vi "Edit Structure.vi"(4 "EOH":u8, 5 "Edit structure":bool, 6 "No. of Bytes":u16, 7 "Channel ID":enum16{""}(ring), 8 "Message ID":u8, 9 "SOH":u8, 11 "MulticolumnListbox in":refnum<vi>) -> ()   [LabVIEW 2020]
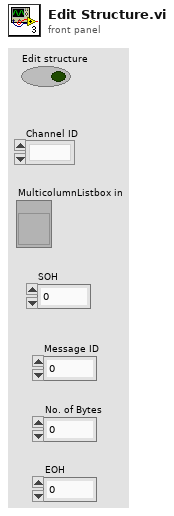
[diagram p1: front panel]
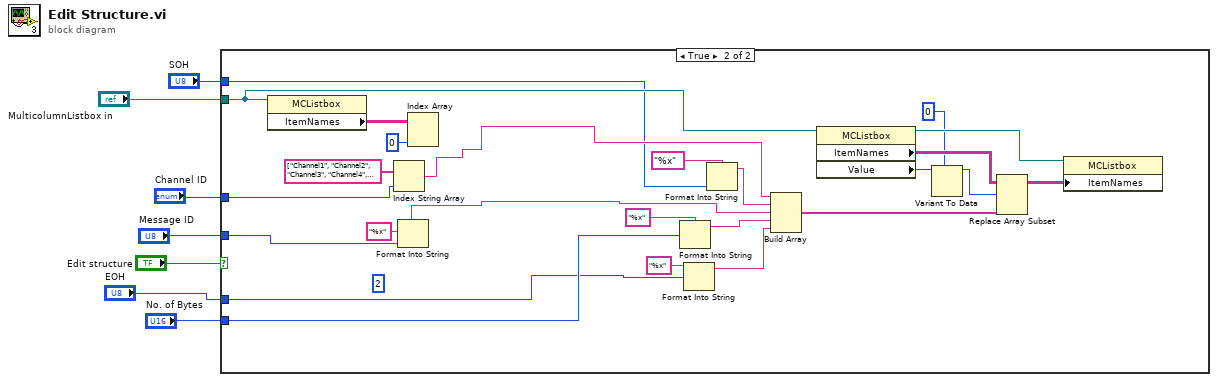
[diagram p0: block diagram]
diagram:
  n1 = case shown="True" "Edit structure" {
    tunnel: "MulticolumnListbox in" -> [_ w27]
    tunnel: "Channel ID" -> [_ w22]
    tunnel: "Message ID" -> [_ w21]
    tunnel: "SOH" -> [_ w25]
    tunnel: "No. of Bytes" -> [_ w24]
    tunnel: "EOH" -> [_ w23]
    frame False {
    }
    frame True {
      (unwired) 2 ("disabled index (col)")
      n2 = property class="MCListbox"(reference=w27) -> ("ItemNames"=w30:string[][])  [unwired: 1 in, 2 out]
      n3 = Index String Array(1:w22, 2:string[] ["Channel1", "Channel2", "Channel3", "Channel4", "Channel5", "Channel6", "Channel7", "Channel8"] ("string array")) -> (0:w29:string)  [unwired: 1 in]
      n4 = Format Into String(format string="%x", w21) -> (resulting string=w28:string)  [unwired: 2 in, 1 out]
      n5 = Index Array(array=w30, index (col)=0 ("disabled index (col)")) -> ()  [unwired: 1 in, 1 out]
      n6 = Format Into String(format string="%x", w24) -> (resulting string=w19:string)  [unwired: 2 in, 1 out]
      n7 = Format Into String(format string="%x", w23) -> (resulting string=w18:string)  [unwired: 2 in, 1 out]
      n8 = Format Into String(format string="%x", w25) -> (resulting string=w20:string)  [unwired: 2 in, 1 out]
      n9 = Build Array(w29, w20, w28, w19, w18) -> (w15:string[])
      n10 = property class="MCListbox"(reference=w27) -> (reference out=w13:refnum<vi>, "ItemNames"=w17:string[][], "Value"=w16:variant)  [unwired: 1 in, 1 out]
      n11 = Variant To Data(type=u32 0, Variant=w16) -> (data=w8:u32)  [unwired: 1 in, 1 out]
      n12 = Replace Array Subset(array=w17, new element=w15, index (row)=w8) -> (w14:string[][])  [unwired: 1 in]
      n13 = property class="MCListbox"(reference=w13, "ItemNames"=w14) -> ()  [unwired: 1 in, 2 out]
    }
  }
